vi "rtp play.vi"(4 "voltage range":dbl, 6 "freq":u32, 7 "rtp stop event ref":refnum<user-event>, 8 "error in (no error)":errorcluster caption="에러 입력(에러 없음)", 10 "waveform data":i8[](array[numeric]), 11 "Haptic IC 입력":refnum<class "Haptic IC.lvclass">) -> (0 "error out":errorcluster caption="에러 출력", 3 "Haptic IC 출력":refnum<class "Haptic IC.lvclass">)   [LabVIEW 2020, in "Haptic IC.lvclass"]
uses:
  Haptic IC.lvclass
  rtp play core.vi
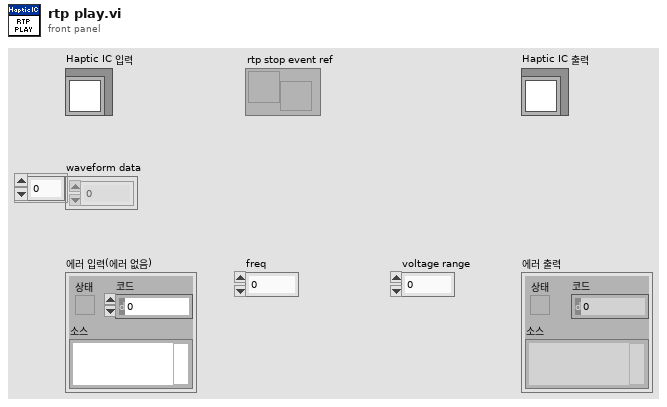
[diagram p1: front panel]
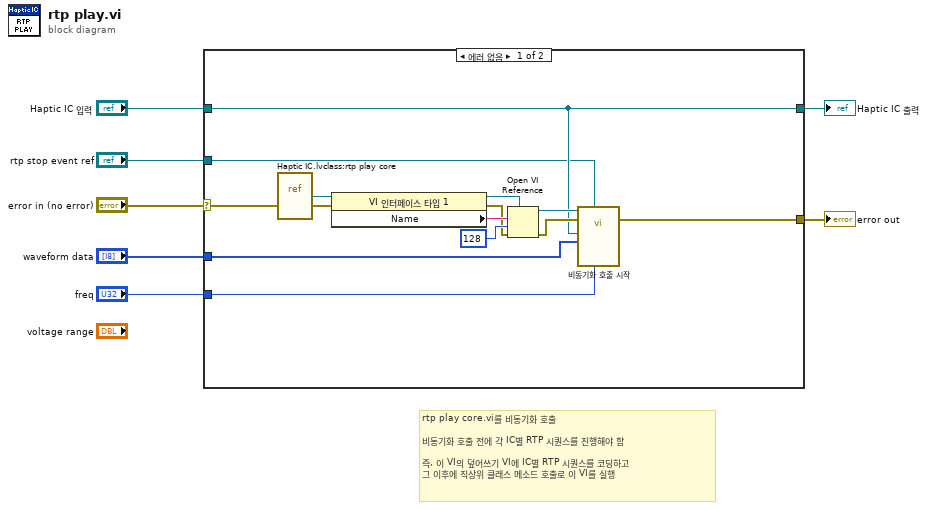
[diagram p0: block diagram]
diagram:
  # "rtp play core.vi를 비동기화 호출\n\n비동기화 호출 전에 각 IC별 RTP 시퀀스를 진행해야 함\n\n즉, 이 VI의 덮어쓰기 VI에 IC별 RTP 시퀀스를 코딩하고\n그 이후에 직상위 클래스 메소드 호출로 이 VI를 실행"
  n1 = case shown="에러 없음" "error in (no error)" {
    selector: "error in (no error)" -> [w9 w22]
    tunnel: [w8 w22] -> w6
    tunnel: [w13 w21] -> w4
    tunnel: "Haptic IC 입력" -> [w13 w21]
    tunnel: "rtp stop event ref" -> [w12 _]
    tunnel: "waveform data" -> [w11 _]
    tunnel: "freq" -> [w10 _]
    frame No Error {
      n2 = vi-ref "Haptic IC.lvclass:rtp play core.vi"() -> (w20:refnum<vi>)
      n3 = property class="VI 인터페이스 타입 1"(reference=w20, error in=w9) -> (reference out=w18:refnum<vi>, error out=w14:errorcluster, "Name"=w19:string)
      n4 = Open VI Reference(type specifier VI Refnum (for type only)=w18, vi path=w19, options=128 ("옵션"), error in (no error)=w14) -> (vi reference=w16:refnum<vi>, error out=w15:errorcluster)  [unwired: 2 in]
      n5 = call-by-ref "비동기화 호출 시작"(reference=w16, error in=w15, "freq"=w10, "rtp stop event ref"=w12, "waveform data"=w11, "Haptic IC 입력"=w13) -> (error out=w8:errorcluster)  [unwired: 6 in, 3 out]
    }
    frame Error {
    }
  }
  "error out" <- w6
  "Haptic IC 출력" <- w4
